vi "Write Contestant Names.vi"(8 "error in (no error)":errorcluster, 10 "Contestant Names":string[](array[string]), 11 "MC Prompt in":refnum<class "MC Prompt.lvclass">) -> (0 "error out":errorcluster, 3 "MC Prompt out":refnum<class "MC Prompt.lvclass">)   [LabVIEW 2024, in "MC Prompt.lvlib" / "MC Prompt.lvclass"]
uses:
  MC Prompt.lvclass
  MC Prompt.lvclass/MC Prompt.ctl
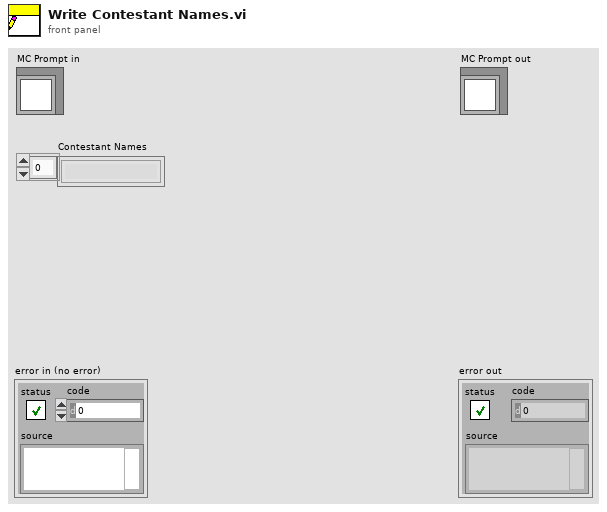
[diagram p1: front panel]
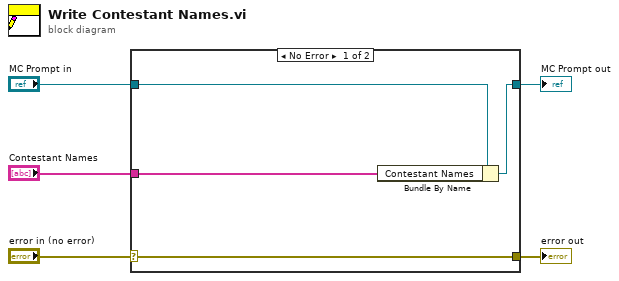
[diagram p0: block diagram]
diagram:
  n1 = case shown="No Error" "error in (no error)" {
    selector: "error in (no error)" -> [w9 w10]
    tunnel: [w9 w10] -> w4
    tunnel: [w7 w11] -> w2
    tunnel: "MC Prompt in" -> [w8 w11]
    tunnel: "Contestant Names" -> [w6 _]
    frame No Error {
      n2 = Bundle By Name(cluster=w8, "Contestant Names"=w6) -> (w7:refnum<class "MC Prompt.lvclass">)
    }
    frame Error {
    }
  }
  "error out" <- w4
  "MC Prompt out" <- w2
